vi "origin_export.vi"(8 "error in (no error)":errorcluster, 9 "Origin File":path, 10 "Book Name":string, 11 "file path (dialog if empty)":path) -> (0 "error out":errorcluster)   [LabVIEW 2013]
uses:
  <vilib>/Utility/file.llb/Read From Spreadsheet File (string).vi
  <vilib>/Utility/file.llb/Read From Spreadsheet File (DBL).vi
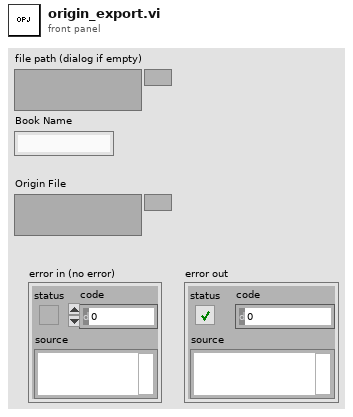
[diagram p1: front panel]
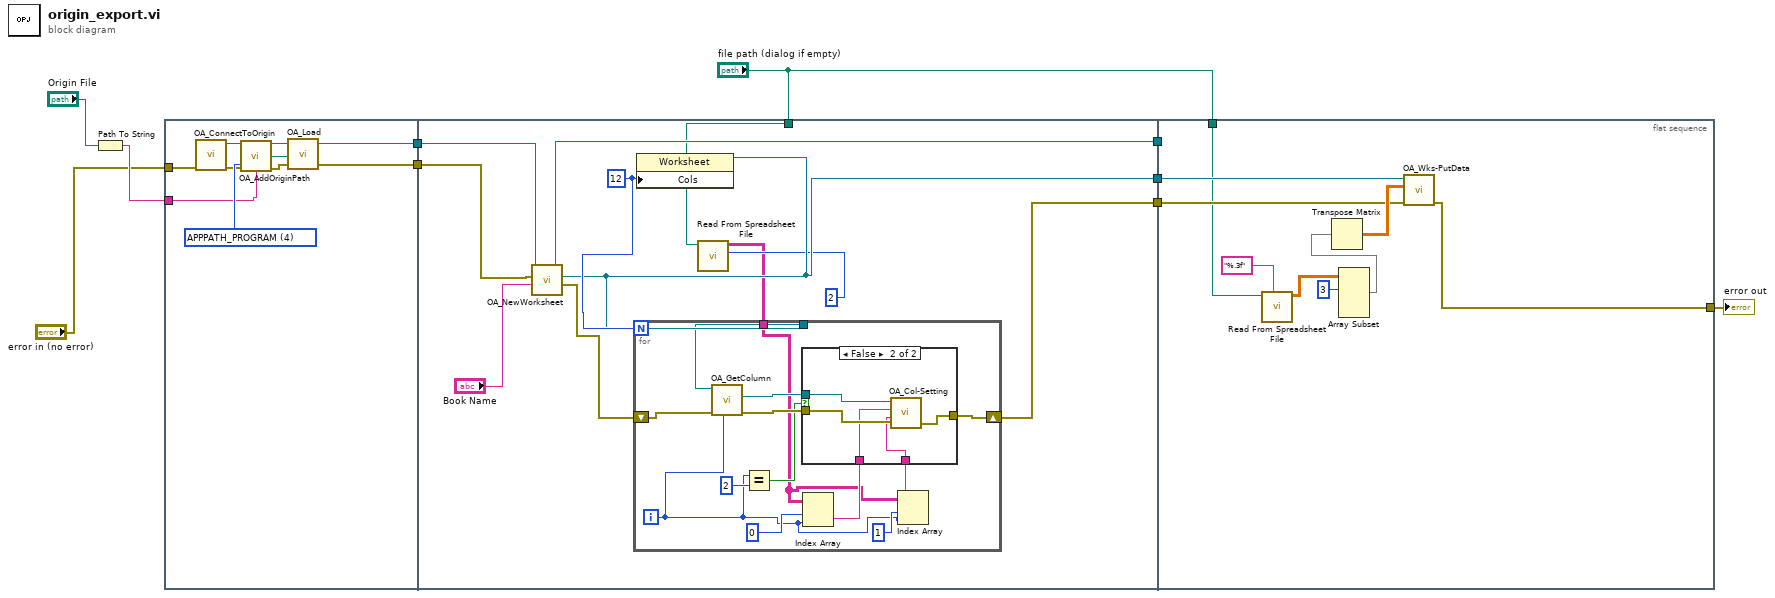
[diagram p0: block diagram]
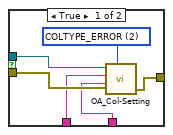
[diagram p2: hidden frame]
diagram:
  n1 = Path To String(path="Origin File") -> (string=w3:string)
  n2 = flat-sequence {
    tunnel: [w14] -> w10
    tunnel: [w13] -> w9
    tunnel: w3 -> [w12]
    tunnel: "error in (no error)" -> [w11]
    tunnel: w10 -> [w30]
    tunnel: w9 -> [w31]
    tunnel: [w28] -> w8
    tunnel: [w25] -> w7
    tunnel: [w24] -> w6
    tunnel: "file path (dialog if empty)" -> [w22]
    tunnel: w8 -> [_]
    tunnel: [w64] -> w1
    tunnel: w7 -> [w58]
    tunnel: w6 -> [w57]
    tunnel: "file path (dialog if empty)" -> [w56]
    frame #0 {
      w19 = 4 items=["APPPATH_USER"=2, "APPPATH_GROUP"=3, "APPPATH_PROGRAM"=4] ("Type")
      n3 = call "OA_ConnectToOrigin.vi"("error in (no error)"=w11) -> ("error out"=w15:errorcluster, "Origin.IOApplication"=w20:refnum<k7>)  [unwired: 7 in]
      n4 = call "OA_AddOriginPath.vi"("Origin.IOApplication"=w20, "error in (no error)"=w15, "Type"=w19, "Filename"=w12) -> ("Origin.IOApplication"=w16:refnum<k7>, "path out"=w18:path, "error out"=w17:errorcluster)  [unwired: 9 in]
      n5 = call "OA_Load.vi"("error in (no error)"=w17, "Path"=w18, "Origin.IOApplication"=w16) -> ("error out"=w14:errorcluster, "Origin.IOApplication"=w13:refnum<k7>)  [unwired: 1 out]
    }
    frame #1 {
      w26 = 12
      n6 = call "OA_NewWorksheet.vi"("Book Name"="Book Name", "error in (no error)"=w30, "Origin.IOApplication"=w31) -> ("error out"=w27:errorcluster, "Origin.Worksheet"=w25:refnum<k7>, "Origin.IOApplication"=w28:refnum<k7>)  [unwired: 4 in]
      n7 = property class="Worksheet"(reference=w25, "Cols"=w26) -> ()  [unwired: 1 in, 2 out]
      n8 = call-poly <vilib>:"Read From Spreadsheet File.vi"("number of rows (all:-1)"=2, "file path (dialog if empty)"=w22) -> ("all rows"=w21:string[][])  [unwired: 5 in, 4 out]
      n9 = for {
        N: w26 -> [_]
        tunnel: w25 -> [w44]
        shift-right: [w41] -> w24
        shift-left: w27 -> [w40]
        tunnel: w21 -> [w35]
        i -> [w32]
        n10 = call "OA_GetColumn.vi"("Column Name/Index"=w32, "error in (no error)"=w40, "Origin.Worksheet"=w44) -> ("error out"=w42:errorcluster, "Origin.Column"=w43:refnum<k7>)  [unwired: 6 in, 1 out]
        n11 = Equal?(x=w32, y=2) -> (x = y?=w38:bool)
        n12 = Index Array(array=w35, index (row)=0 ("disabled index (row)"), index (col)=w32) -> (element=w36:string)
        n13 = Index Array(array=w35, index (row)=1 ("disabled index (col)"), index (col)=w32) -> (element=w34:string)
        n14 = case shown="False" w38 {
          tunnel: w43 -> [w50 w55]
          tunnel: w42 -> [w49 w54]
          tunnel: [w48 w53] -> w41
          tunnel: w36 -> [w46 w52]
          tunnel: w34 -> [w45 w51]
          frame True {
            w47 = 2 items=["COLTYPE_NO_CHANGE"=-1, "COLTYPE_Y"=0, "COLTYPE_NONE"=1, "COLTYPE_ERROR"=2, "COLTYPE_X"=3, "COLTYPE_LABEL"=4, "COLTYPE_Z"=5, "COLTYPE_X_ERROR"=6, "COLTYPE_GROUP"=7, "COLTYPE_SUBJECT"=8] ("Type")
            n15 = call "OA_Col-Setting.vi"("Origin.Column"=w50, "Type"=w47, "LongName"=w46, "Units"=w45, "error in (no error)"=w49) -> ("error out"=w48:errorcluster)  [unwired: 2 in, 1 out]
          }
          frame False {
            n16 = call "OA_Col-Setting.vi"("Origin.Column"=w55, "LongName"=w52, "Units"=w51, "error in (no error)"=w54) -> ("error out"=w53:errorcluster)  [unwired: 3 in, 1 out]
          }
        }
      }
    }
    frame #2 {
      n17 = call-poly <vilib>:"Read From Spreadsheet File.vi"("format (%.3f)"="%.3f", "file path (dialog if empty)"=w56) -> ("all rows"=w61:dbl[][])  [unwired: 5 in, 4 out]
      n18 = Array Subset(array=w61, index (row)=3 ("index")) -> (w59:dbl[][])  [unwired: 3 in]
      n19 = Transpose Matrix(1:w59) -> (0:w62:dbl[][])
      n20 = call "OA_Wks-PutData.vi"("error in (no error)"=w57, "2d Data"=w62, "Origin.Worksheet"=w58) -> ("error out"=w64:errorcluster)  [unwired: 2 in, 2 out]
    }
  }
  "error out" <- w1
